vi "客服端INI.vi"(0 "客服端参数":cluster{"本机端口":u16, "主机 IP":string, "主机端口":u16}={"本机端口"=0, "主机 IP"="0", "主机端口"=0}) -> (14 "连接ID":refnum<k5>, 16 "可用？":bool)   [LabVIEW 2019, in "MainPage.lvlib" / "MainPage.lvclass"]
uses:
  MainPage.lvclass
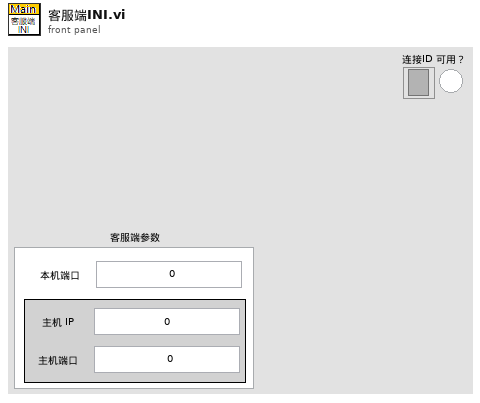
[diagram p1: front panel]
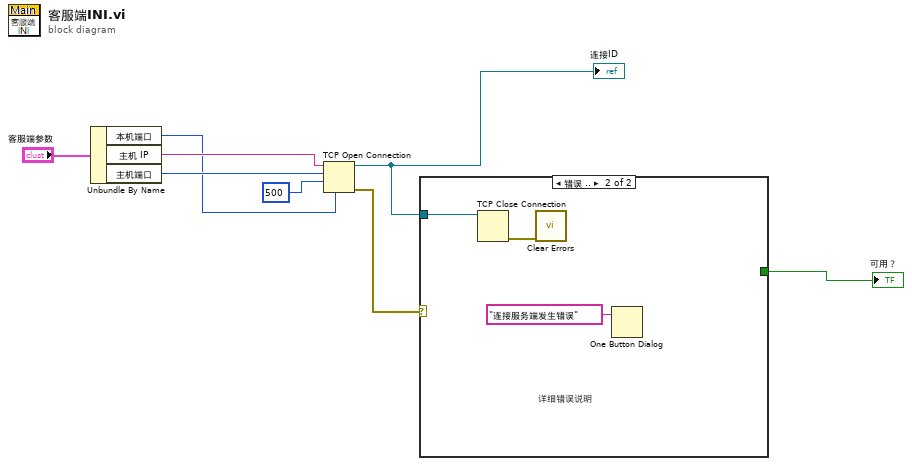
[diagram p0: block diagram]
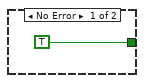
[diagram p2: hidden frame]
diagram:
  n1 = Unbundle By Name("客服端参数") -> ("本机端口"=w5:u16, "主机 IP"=w7:string, "主机端口"=w6:u16)
  n2 = TCP Open Connection(address=w7, remote port or service name=w6, timeout ms (60000)=500 ("超时毫秒(60000)"), local port=w5) -> (connection ID=w1:refnum<k5>, error out=w3:errorcluster)  [unwired: 1 in]
  "连接ID" <- w1
  n3 = case shown="错误 .." w3 {
    tunnel: [TRUE _] -> w2
    tunnel: w1 -> [_ w10]
    frame No Error {
    }
    frame Error {
      # "详细错误说明"
      n4 = TCP Close Connection(connection ID=w10) -> (error out=w11:errorcluster)  [unwired: 2 in, 1 out]
      n5 = call <vilib>:"Clear Errors.vi"("error in (no error)"=w11) -> ()  [unwired: 5 in, 2 out]
      n6 = One Button Dialog(message="连接服务端发生错误" ("消息")) -> ()  [unwired: 1 in, 1 out]
    }
  }
  "可用？" <- w2
